vi "9159 FPGA VI.vi"() -> ()   [LabVIEW 2017]
uses:
  <vilib>/Platform/TimedLoop/XDataNode/timing_clust.ctl
  <vilib>/Platform/TimedLoop/XDataNode/nitl_modes.ctl
  <vilib>/Platform/TimedLoop/XDataNode/wakeup.ctl
  <vilib>/rvi/Emulation/niFpgaGetClockAttributes.vi
  <vilib>/rvi/Emulation/niFpgaSctlEmulationGetInTimedLoop.vi
  <vilib>/rvi/Emulation/niFpgaEmulationReportErrorSimple.vi
  <vilib>/rvi/eio/common/nirviEmuTemplateMethod_errors.vi
  <vilib>/rvi/Emulation/niFpgaEmulationIsFPGAContextNoSignature.vi
  <vilib>/rvi/errors/niFpgaSetErrorForExecOnDevCompSimple.vi
  <vilib>/rvi/eio/common/nirviEmuReportErrorAndStop.vi
  <vilib>/rvi/DataTransferAndStorage/Container/Common/niFpgaContainerGetUniqueNameForEmu.vi
  <vilib>/rvi/FIFO/Fifo_Resource/nirvififoEmulationSetSize.vi
  <vilib>/rvi/FIFO/Fifo_Resource/nirviFifoEmulationQueueMgr.vi
  <instcachedir>/0/nirviFifoEmulationQueueMgr_E5CAEC123FF24DC58D834DCA3CDAA9B5.lvgen/nirviFifoEmulationQueueMgr_E5CAEC123FF24DC58D834DCA3CDAA9B5_008.vi
  <vilib>/rvi/FIFO/Fifo_Resource/nirvififoEmulationDetermineInputValidOut.vi
  <vilib>/rvi/FIFO/Fifo_Resource/nirvififoEmulationCreateLock.vi
  <vilib>/rvi/Emulation/niFpgaProcessEmulError.vi
  <vilib>/rvi/FIFO/Fifo_Resource/nirvififoEmulationObtainLock.vi
  <vilib>/rvi/FIFO/Fifo_Resource/nirvififoEmulationReleaseLock.vi
  <vilib>/rvi/occurrence/nirviWaitOnOccurrenceBase.vi
  <vilib>/rvi/errors/nirviReportUnexpectedCaseInternalError.vi
  <vilib>/rvi/errors/nirviReportUnexpectedCaseInternalError (U32).vi
  <vilib>/rvi/Emulation/niFpgaCriticalErrorInLSC.vi
  <vilib>/rvi/interface/RandomDataEmulation/niFpgaRandomDataHandleErrors.vi
  <vilib>/Utility/error.llb/Clear Errors.vi
  <vilib>/eio/EIONode/EIONode.xnode
  <vilib>/rvi/DataTransferAndStorage/Container/XNode/niFpgaContainer.xnode
  <vilib>/rvi/FIFO/Fifo_Resource/nirvififoEmulationWrite.vi
  <vilib>/rvi/interface/RandomDataEmulation/nirviRandomDataFpgaReadWriteTemplate.vi
  <vilib>/Platform/TimedLoop/XDataNode/XDataNode.xnode
  <vilib>/rvi/FIFO/Fifo_Resource/nirvififoEmulationRead.vi
  <vilib>/Platform/TimedLoop/XDataNode/XDNodeRunTimeDep.lvlib
panel:
  out "ArbDataLoop_TimedOut":bool
  in  "SlowIOScanLoop_Toggle":bool
  out "ArbFIFO_Done":bool
  in  "ArbFIFO_Sample_Value":u64=555
  in  "ArbFIFO_Read_Size_Samples":i16=1000
  in  "Trigger_ArbFIFO_Bool":bool
  out "Mod3_AI15_I32":i32
  out "Mod3_AI14_I32":i32
  out "Mod3_AI13_I32":i32
  out "Mod3_AI12_I32":i32
  out "Mod3_AI11_I32":i32
  out "Mod3_AI10_I32":i32
  out "Mod3_AI9_I32":i32
  out "Mod3_AI8_I32":i32
  out "Mod3_AI7_I32":i32
  out "Mod3_AI6_I32":i32
  out "Mod3_AI5_I32":i32
  out "Mod3_AI4_I32":i32
  out "TargetToHostLoopIterCount":i32
  out "TargetToHostLoopTimedOut":bool
  out "Mod6_U32":u32
  out "Mod5_U32":u32
  out "Mod2_U8":u8
  in  "Mod11_U32":u32
  in  "Mod10_U32":u32
  in  "Mod9_U32":u32
  in  "Mod7_U32":u32
  in  "SlowDOLoop_Rate_us":u32=10000 caption="Count(uSec)"
  out "SlowDOLoop_Duration_ticks":u32
  in  "FastAILoop_Rate_us":u32=1000 caption="Count(uSec)"
  out "FastAILoop_Duration_ticks":u32
  out "Mod3_AI3_I32":i32
  out "Mod3_AI2_I32":i32
  out "Mod3_AI1_I32":i32
  out "Mod3_AI0_I32":i32
  out "SlowIOScanLoopTimedOut":bool
  out "SlowScanLoop_Duration_ticks":u32
  in  "SlowScanLoop_Rate_us":u32=10000 caption="Count(uSec)"
  in  "FastDO_U8":u8
  out "FastDI_U8":u8
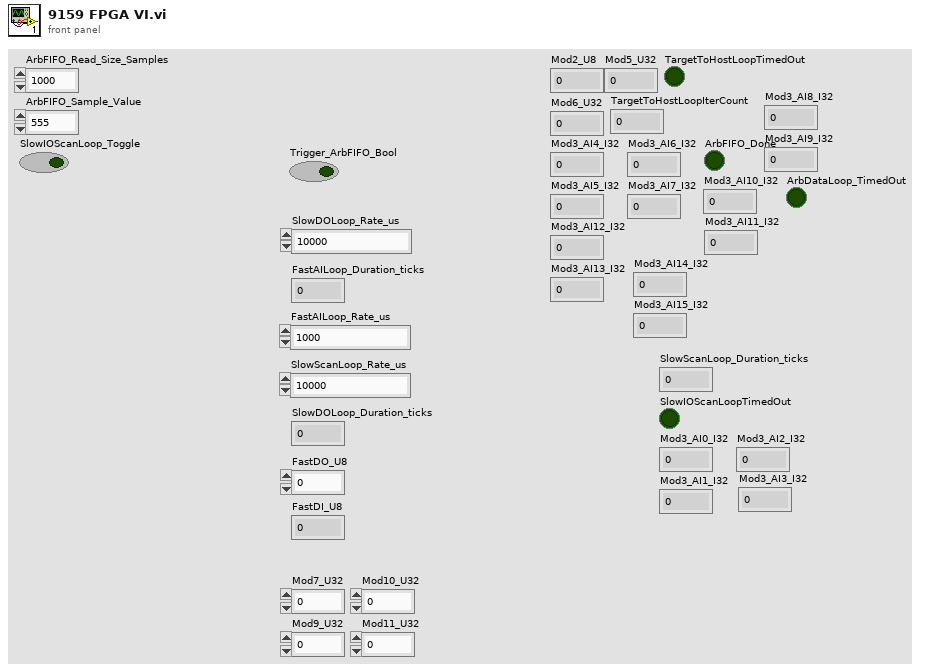
[diagram p1: front panel]
types:
  T1 = typedef "XDNodeRunTimeDep.lvlib/timing_clust.ctl" = cluster{"Expected End [f-1]":u64, "Actual End [f-1]":u64, "Finished Late? [f-1]":bool, "Expected End [i-1]":u64, "Actual End [i-1]":u64, "Finished Late? [i-1]":bool, "Expected Start [i]":u64, "Actual Start [i]":u64, "Expected Start [f]":u64, "Actual Start [f]":u64, "Source Name":string, "Structure Name":string, "Period":i64, "Deadline":i64, "Offset":i64, "Start":i64, "Priority":i32, "Timeout":i32, "Mode":T2, "Wakeup Reason":T3, "Error":errorcluster, "Source Type":string, "Secondary Source Type":string, "Global End Time":u64, "Global Start Time":u64, "Frame Duration":u64, "Iteration Duration":u64, "Assigned CPU":i32, "I/O Scan Engine Mode":u32}
  T2 = typedef "XDNodeRunTimeDep.lvlib/nitl_modes.ctl" = enum32{"No Change", "Process missed periods, maintain original phase", "Discard missed periods, maintain original phase", "Process missed periods, ignore original phase", "Discard missed periods, ignore original phase"}
  T3 = typedef "XDNodeRunTimeDep.lvlib/wakeup.ctl" = enum32{"Normal", "Aborted", "Asynchronous wakeup", "Timing source error", "Timed loop error", "Timeout"}
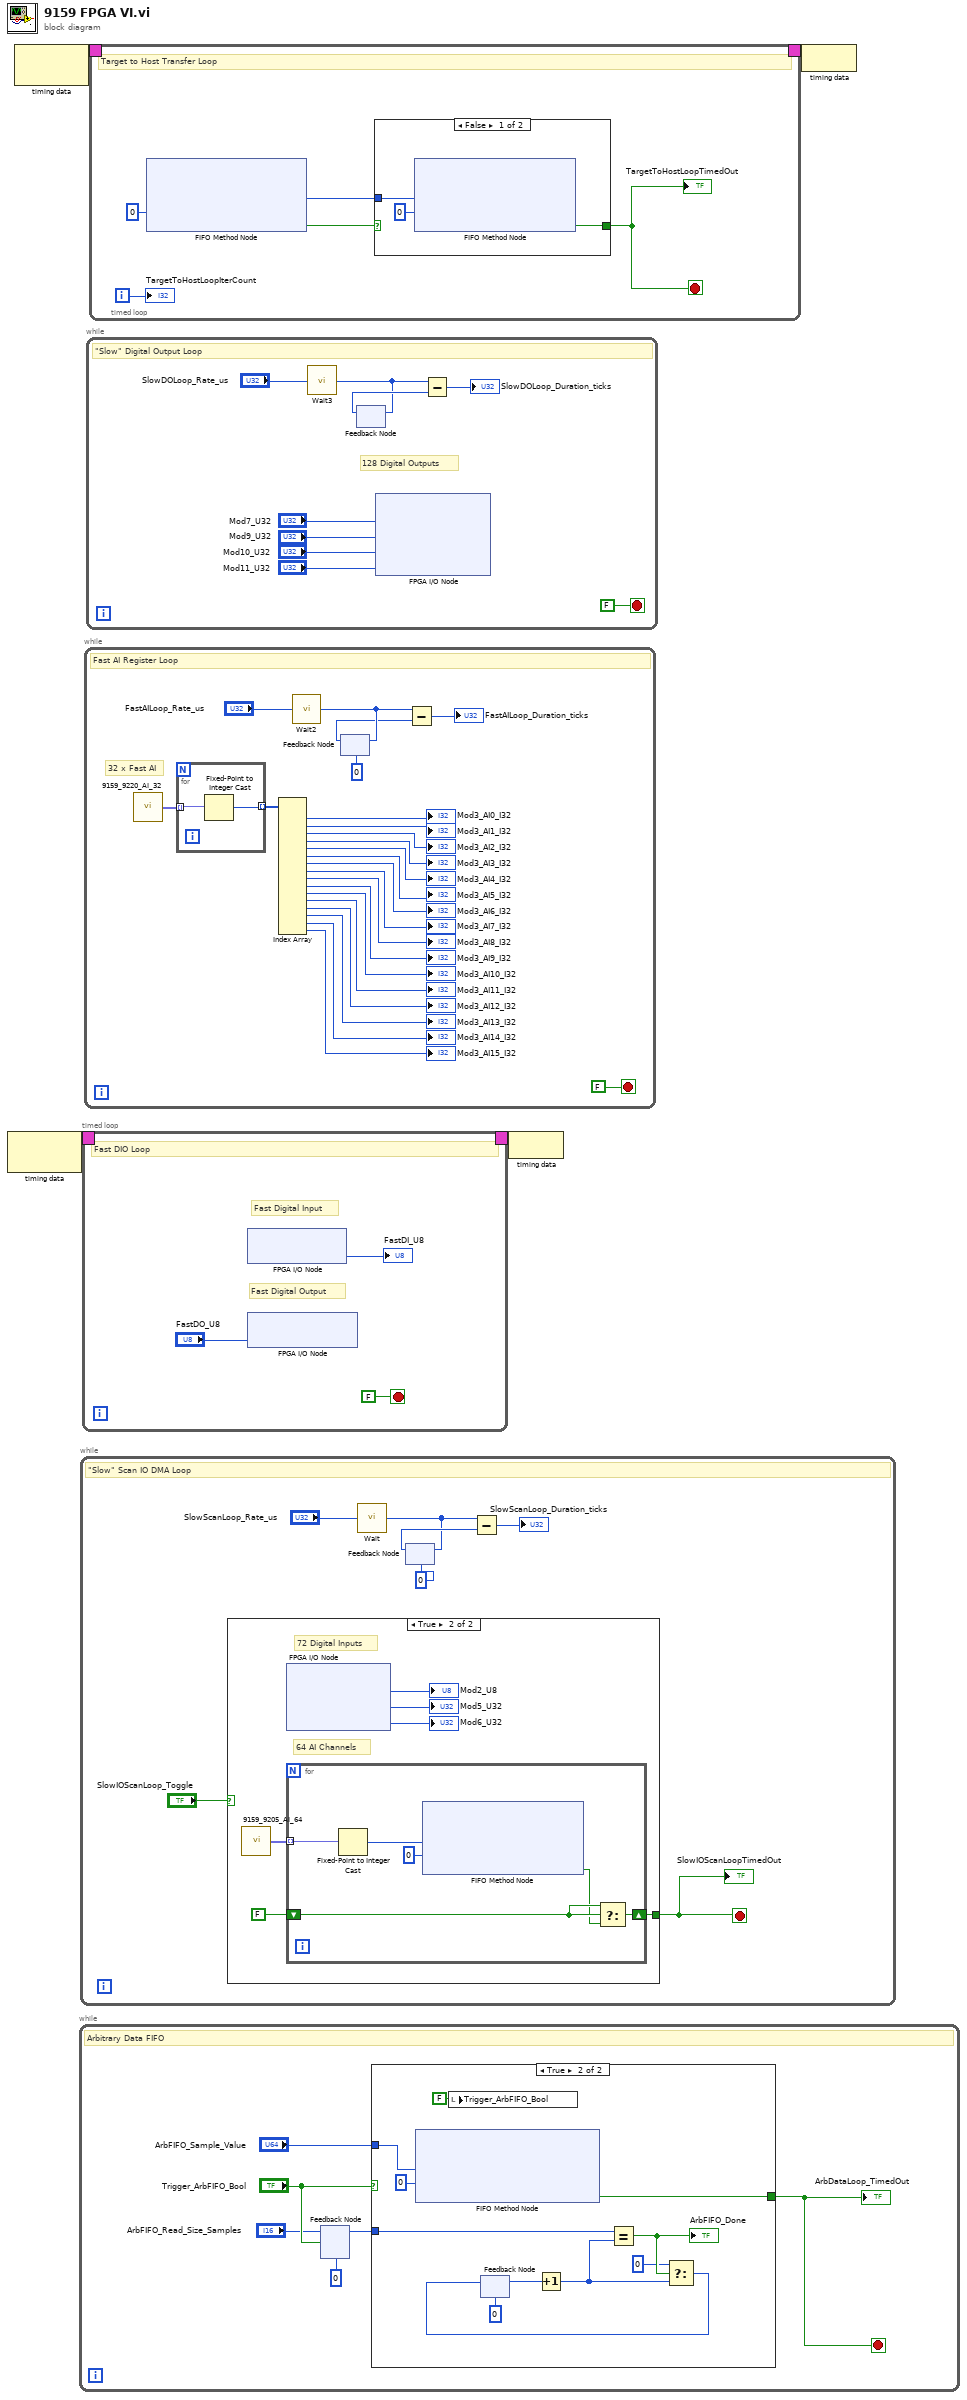
[diagram p0: block diagram]
diagram:
  n1 = node-c288() -> (w2:T1)  [unwired: 1 in]
  n2 = node-c288() -> (w4:T1)  [unwired: 1 in]
  n3 = while {
    stop <- w9 stop-if-true
    # "Arbitrary Data FIFO"
    n4 = feedback-in #1("ArbFIFO_Read_Size_Samples", "Trigger_ArbFIFO_Bool") -> ()
    n5 = feedback #1(i16 0 ("Timeout")) -> (w7:i16)
    n6 = case shown="True" "Trigger_ArbFIFO_Bool" {
      tunnel: "ArbFIFO_Sample_Value" -> [_ w18]
      tunnel: [_ w21] -> w9
      tunnel: w7 -> [_ w15]
      frame False {
      }
      frame True {
        n7 = xnode ("FIFO Method Node")("Element"=w18, "Timeout"=0) -> ("Timed Out?"=w21:bool)  [unwired: 1 in, 1 out]
        n8 = local write "Trigger_ArbFIFO_Bool"(FALSE) -> ()
        n9 = feedback #2(i16 0 ("Timeout")) -> (w16:i16)
        n10 = Increment(x=w16) -> (x+1=w12:i16)
        n11 = Equal?(x=w15, y=w12) -> (x = y?=w14:bool)
        "ArbFIFO_Done" <- w14
        n12 = Select(t=i16 0 ("Timeout"), s=w14, f=w12) -> (s? t:f=w11:i16)
        n13 = feedback-in #2(w11) -> ()
      }
    }
    "ArbDataLoop_TimedOut" <- w9
  }
  n14 = while {
    stop <- w28 stop-if-true
    # "\"Slow\" Scan IO DMA Loop"
    n15 = case shown="True" "SlowIOScanLoop_Toggle" {
      tunnel: [_ w34] -> w28
      frame False {
      }
      frame True {
        # "64 AI Channels"
        # "72 Digital Inputs"
        n16 = call "9159_9205_AI_64.vi"() -> ("Array"=w29:fxp<+/-,26,5>[])  [unwired: 1 in]
        n17 = xnode "FPGA I/O Node"() -> ("Mod2/DI7:0"=→"Mod2_U8":u8, "Mod5/DI31:0"=→"Mod5_U32":u32, "Mod6/DI31:0"=→"Mod6_U32":u32)  [unwired: 3 in, 3 out]
        n18 = for {
          shift-right: [w38] -> w34
          shift-left: FALSE ("Timed Out?") -> [w40]
          tunnel: w29 -> [w37] mode=indexing
          n19 = Fixed-Point to Integer Cast(1:w37) -> (0:w36:i32)
          n20 = xnode ("FIFO Method Node")("Element"=w36, "Timeout"=0) -> ("Timed Out?"=w39:bool)  [unwired: 1 in, 1 out]
          n21 = Select(t=w40, s=w40, f=w39) -> (s? t:f=w38:bool)
        }
      }
    }
    "SlowIOScanLoopTimedOut" <- w28
    n22 = call "Wait"("Count(uSec)"="SlowScanLoop_Rate_us") -> ("Tick Count(uSec)"=w24:u32)
    n23 = feedback #3(u32 0 ("Tick Count(uSec)")) -> (w25:u32)
    n24 = feedback-in #3(w24) -> ()
    n25 = Subtract(x=w24, y=w25) -> (x-y=→"SlowScanLoop_Duration_ticks":u32)
  }
  n26 = timed-loop {
    timing: w2 -> [_]
    timing-out: [_] -> w1
    stop <- FALSE stop-if-true
    # "Fast Digital Output"
    # "Fast Digital Input"
    # "Fast DIO Loop"
    n27 = xnode "FPGA I/O Node"() -> ("Mod8/DI7:0"=→"FastDI_U8":u8)  [unwired: 1 in, 1 out]
    n28 = xnode "FPGA I/O Node"("Mod12/DO7:0"="FastDO_U8") -> ()  [unwired: 1 in, 1 out]
  }
  n29 = while {
    stop <- FALSE stop-if-true
    # "32 x Fast AI"
    # "Fast AI Register Loop"
    n30 = call "9159_9220_AI_32.vi"() -> ("Array"=w68:fxp<+/-,24,5>[])  [unwired: 1 in]
    n31 = for {
      tunnel: w68 -> [w71] mode=indexing
      tunnel: [w70] -> w67 mode=indexing
      n32 = Fixed-Point to Integer Cast(1:w71) -> (0:w70:i32)
    }
    n33 = Index Array(array=w67) -> (element #1=→"Mod3_AI0_I32":i32, element #2=→"Mod3_AI1_I32":i32, element #3=→"Mod3_AI2_I32":i32, element #4=→"Mod3_AI3_I32":i32, element #5=→"Mod3_AI4_I32":i32, element #6=→"Mod3_AI5_I32":i32, element #7=→"Mod3_AI6_I32":i32, element #8=→"Mod3_AI7_I32":i32, element #9=→"Mod3_AI8_I32":i32, element #10=→"Mod3_AI9_I32":i32, element #11=→"Mod3_AI10_I32":i32, element #12=→"Mod3_AI11_I32":i32, element #13=→"Mod3_AI12_I32":i32, element #14=→"Mod3_AI13_I32":i32, element #15=→"Mod3_AI14_I32":i32, element #16=→"Mod3_AI15_I32":i32)  [unwired: 16 in]
    n34 = call "Wait2"("Count(uSec)"="FastAILoop_Rate_us") -> ("Tick Count(uSec)"=w61:u32)
    n35 = feedback #4(u32 0 ("Tick Count(uSec)")) -> (w60:u32)
    n36 = feedback-in #4(w61) -> ()
    n37 = Subtract(x=w61, y=w60) -> (x-y=→"FastAILoop_Duration_ticks":u32)
  }
  n38 = while {
    stop <- FALSE stop-if-true
    # "128 Digital Outputs"
    # "\"Slow\" Digital Output Loop"
    n39 = call "Wait3"("Count(uSec)"="SlowDOLoop_Rate_us") -> ("Tick Count(uSec)"=w78:u32)
    n40 = feedback #5() -> (w79:u32)  [unwired: 1 in]
    n41 = feedback-in #5(w78) -> ()
    n42 = xnode "FPGA I/O Node"("Mod7/DO31:0"="Mod7_U32", "Mod9/DO31:0"="Mod9_U32", "Mod10/DO31:0"="Mod10_U32", "Mod11/DO31:0"="Mod11_U32") -> ()  [unwired: 4 in, 4 out]
    n43 = Subtract(x=w78, y=w79) -> (x-y=→"SlowDOLoop_Duration_ticks":u32)
  }
  n44 = timed-loop {
    timing: w4 -> [_]
    timing-out: [_] -> w3
    i -> [w81]
    stop <- w82 stop-if-true
    # "Target to Host Transfer Loop"
    n45 = xnode ("FIFO Method Node")("Timeout"=0) -> ("Element"=w83:i32, "Timed Out?"=w85:bool)  [unwired: 1 in, 1 out]
    n46 = case shown="False" w85 {
      tunnel: w83 -> [w88 _]
      tunnel: [w86 _] -> w82
      frame False {
        n47 = xnode ("FIFO Method Node")("Element"=w88, "Timeout"=0) -> ("Timed Out?"=w86:bool)  [unwired: 1 in, 1 out]
      }
      frame True {
      }
    }
    "TargetToHostLoopTimedOut" <- w82
    "TargetToHostLoopIterCount" <- w81
  }
  n48 = node-c288(w1) -> ()
  n49 = node-c288(w3) -> ()
